vi "foorloop2.vi"() -> ()   [LabVIEW 2020]
panel:
  in  "Numeric 2":i32
  out "x":dbl
  out "Numeric":i32
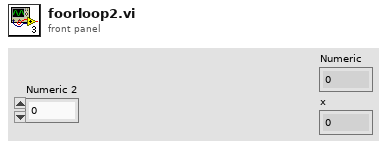
[diagram p1: front panel]
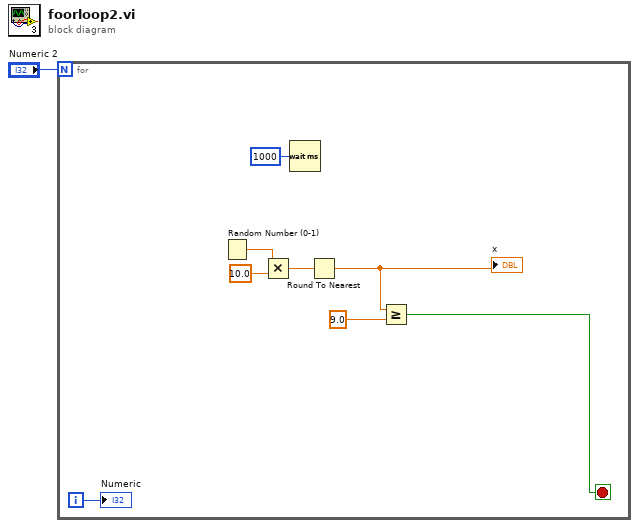
[diagram p0: block diagram]
diagram:
  n1 = for {
    N: "Numeric 2" -> [_]
    i -> [w9]
    stop <- w2 stop-if-true
    n2 = Random Number (0-1)() -> (number: 0 to 1=w8:dbl)
    n3 = Multiply(x=w8, y=10.0) -> (x*y=w5:dbl)
    n4 = Wait (ms)(milliseconds to wait=u32 1000) -> ()  [unwired: 1 out]
    n5 = Round To Nearest(number=w5) -> (nearest integer value=w4:dbl)
    "x" <- w4
    n6 = Greater Or Equal?(x=w4, y=9.0) -> (x >= y?=w2:bool)
    "Numeric" <- w9
  }
